vi "RenameTable.vi"(9 "OldTableName":string, 10 "NewTableName":string, 11 "Path":path) -> (1 "OK？":bool, 2 "Table Name":string, 3 "Path":path)   [LabVIEW 2017, in "SQLite.lvlib"]
uses:
  SQLite.lvlib
  Core/Tables/SQLite_Rename Table.vi
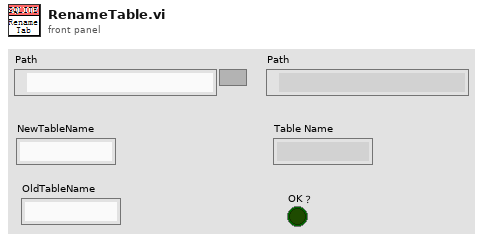
[diagram p1: front panel]
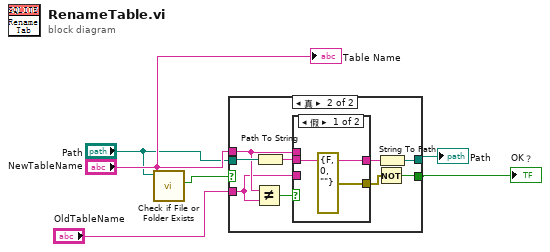
[diagram p0: block diagram]
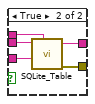
[diagram p3: hidden frame]
diagram:
  n1 = call <vilib>:"Check if File or Folder Exists.vi"("path"="Path") -> ("file or folder exists?"=w2:bool)  [unwired: 8 in, 2 out]
  n2 = case shown="真" w2 {
    selector: w2 -> [w7 _]
    tunnel: "Path" -> [w8 w17]
    tunnel: "NewTableName" -> [_ w10]
    tunnel: [w8 w16] -> w1
    tunnel: [w7 w14] -> w3
    tunnel: "OldTableName" -> [_ w9]
    frame False {
    }
    frame True {
      n3 = Not Equal?(x=w10, y=w9) -> (x != y?=w12:bool)
      n4 = Path To String(path=w17) -> (string=w11:string)
      n5 = case shown="假" w12 {
        tunnel: [w19 w24] -> w15
        tunnel: [errorcluster {"status"=FALSE, "code"=0, "source"=""} ("错误常量") w23] -> w13
        tunnel: w10 -> [_ w22]
        tunnel: w11 -> [w19 w21]
        tunnel: w9 -> [_ w20]
        frame False {
        }
        frame True {
          n6 = call-poly "SQLite_Table.vi"("DB Path"=w21, "Table Name"=w20, "New Table  Name"=w22) -> ("DB Path Out"=w24:string, "error out"=w23:errorcluster)  [unwired: 5 in, 1 out]
        }
      }
      n7 = Not(x=w13) -> (.not. x?=w14:bool)
      n8 = String To Path(string=w15) -> (path=w16:path)
    }
  }
  "OK？" <- w3
  "Path" <- w1
  "Table Name" <- "NewTableName"
